vi "ROI ScopeTrace.vi"(10 "SignalStart":dbl, 11 "raw data":T1) -> (3 "data out":T1)   [LabVIEW 2020]
uses:
  General GUIs/Device GUIs/GUI_Scopes/scopeTrace_TypDef.ctl
panel:
  out "data out":i16[](array[numeric])
  out "fractional index or x":dbl
  out "time axis":dbl[](array[numeric])
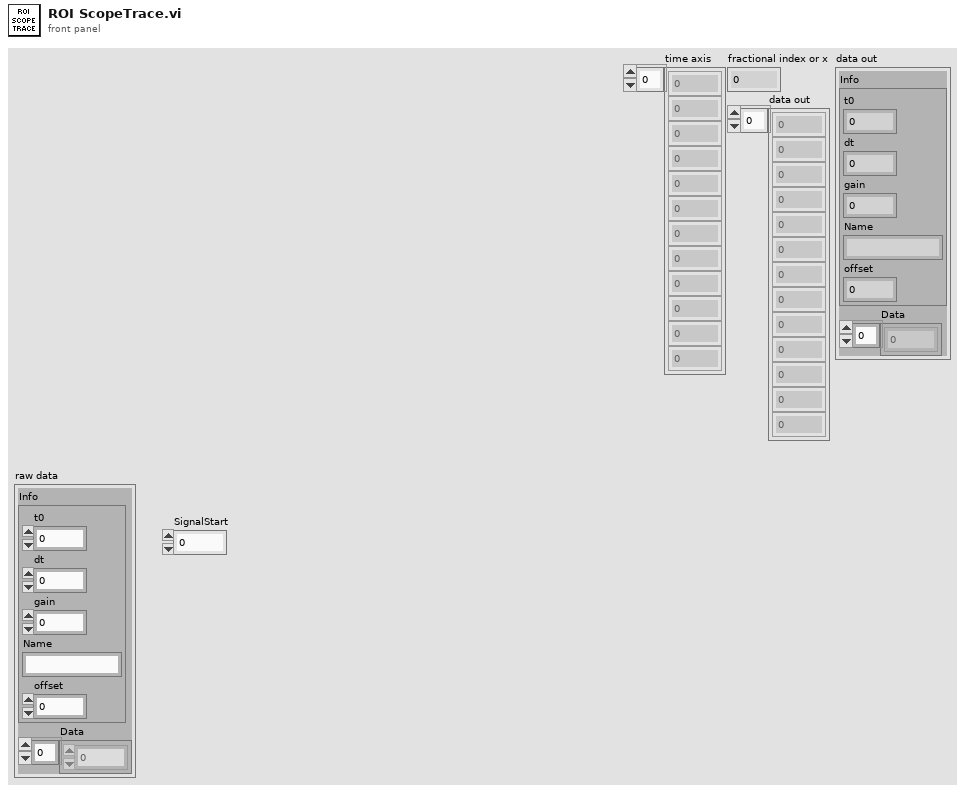
[diagram p1: front panel]
types:
  T1 = typedef "scopeTrace_TypDef.ctl" = cluster{"Info":cluster{"t0":dbl, "dt":dbl, "gain":dbl, "Name":string, "offset":dbl}, "Data":i16[]}
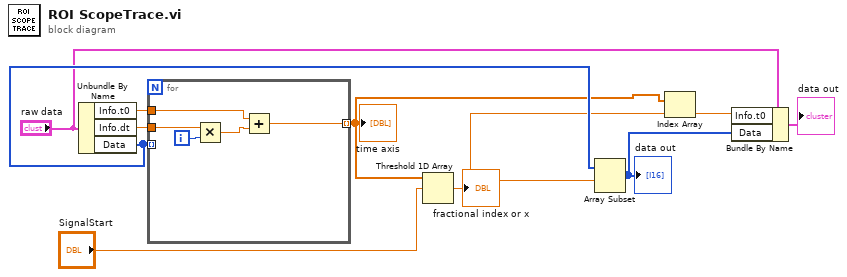
[diagram p0: block diagram]
diagram:
  n1 = Unbundle By Name("raw data") -> ("Info.t0"=w10:dbl, "Info.dt"=w9:dbl, "Data"=w7:i16[])
  n2 = for {
    tunnel: w7 -> [_] mode=indexing
    tunnel: w10 -> [w12]
    tunnel: w9 -> [w14]
    tunnel: [w11] -> w5 mode=indexing
    i -> [w15]
    n3 = Multiply(x=w14, y=w15) -> (x*y=w13:dbl)
    n4 = Add(x=w12, y=w13) -> (x+y=w11:dbl)
  }
  "time axis" <- w5
  n5 = Threshold 1D Array(2:"SignalStart", 3:w5) -> (0:w4:dbl)  [unwired: 1 in]
  "fractional index or x" <- w4
  n6 = Array Subset(array=w7, index=w4) -> (w1:i16[])  [unwired: 1 in]
  "data out" <- w1
  n7 = Index Array(array=w5, index=w4) -> (element=w3:dbl)
  n8 = Bundle By Name(cluster="raw data", "Info.t0"=w3, "Data"=w1) -> (→"data out":T1)
